vi "691E_Global.vi"() -> ()   [LabVIEW 2020]
uses:
  Controls/691E_SET_DI.ctl
  Controls/1357E_DOI_DIO.ctl
  <vilib>/picture/picture.llb/imagedata.ctl
panel:
  out "Dutycycle Message":string
  out "Test Name 2":string
  out "Test Name":string
  out "Correction":T1
  out "Profile Image":picture
  out "FID_Comm":refnum<visa-resource-name>
  in  "Segment":dbl
  out "DPS Fault Bypass?":bool
  in  "PID POINT":dbl
  out "BCK_IMG":T2
  in  "Physical Values_BCK":dbl[][](array[numeric])
  out "In Limits?_Bck":bool[](array[boolean])
  out "DIO Out (16)":bool[](array[boolean])
  out "DO_Ref":refnum<vi>
  in  "PLC IP Address":string
  # "Rhytron Controls"
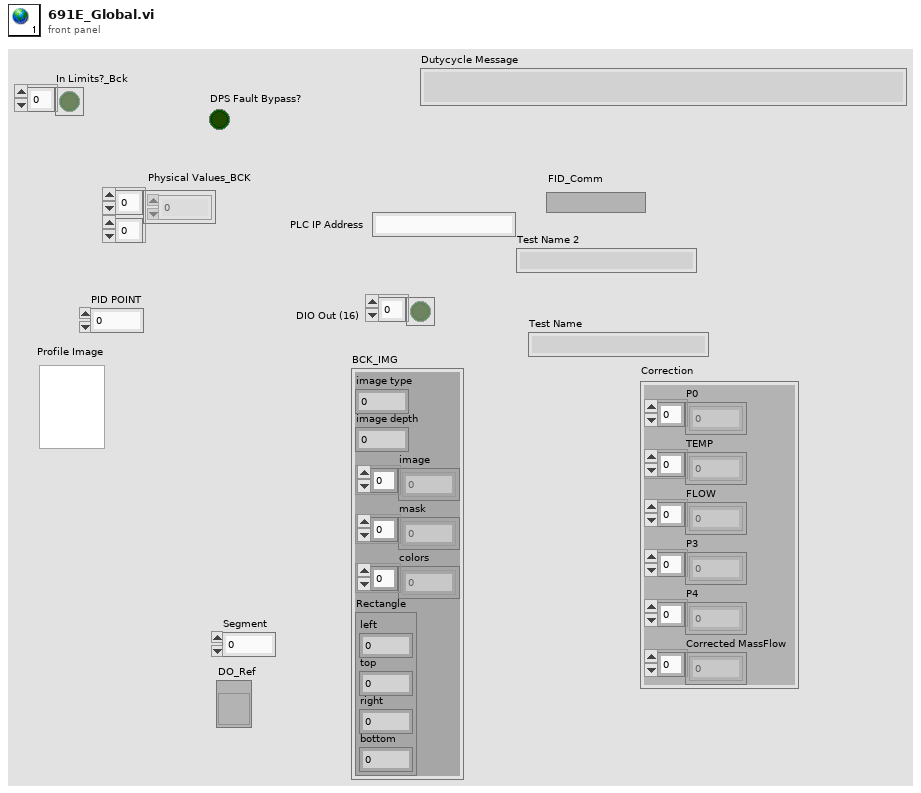
[diagram p1: front panel]
types:
  T1 = cluster{"P0":dbl[], "TEMP":dbl[], "FLOW":dbl[], "P3":dbl[], "P4":dbl[], "Corrected MassFlow":dbl[]}
  T2 = typedef "imagedata.ctl" = cluster{"image type":i32, "image depth":i32, "image":u8[], "mask":u8[], "colors":u32[], "Rectangle":cluster{"left":i16, "top":i16, "right":i16, "bottom":i16}}
diagram:
